vi "Sensor-Resistance-Sampling_withg_SMU1ar.vi"(1 "hold time (sec)":dbl=10.0 format="%#_13g", 2 "Gate step - extra milliseconds to wait":u32=20000, 3 "Current through sensor (A)":dbl format="%#_13g", 4 "Number of times measurement is done":i32=7, 6 "Number of heater steps":i32=7, 7 "Heater Step (V)":dbl=3.3) -> ()   [LabVIEW 2016]
uses:
  <vilib>/Utility/file.llb/Write To Spreadsheet File (DBL).vi
  <vilib>/Utility/file.llb/Read From Spreadsheet File (DBL).vi
  Driver/New driver/Agilent 415X Series.lvlib
panel:
  in  "Gate Step":dbl=-6.0
  in  "Gate Start":dbl format="%#_13g"
  in  "number of samples per heater step":i32=10
  out "error out":errorcluster
  out "Voltage across heater (VSU 1 and SMU4)":dbl[][](graph)
  out "Voltage measured between SMU1 (Common) and SMU2":dbl[](graph)
  out "SPA VISA resource name":refnum<visa-resource-name>
  in  "1. SPA VISA resource name":refnum<visa-resource-name>="GPIB0::14::INSTR"
  in  "error in (no error)":errorcluster
  # "2. Heater Parameters"
  # "3. Repeat Entire Cycle"
  # "4. Timings \n(Should be same as those when sampling Thermopower)"
  # "5. Other measurement parameters"
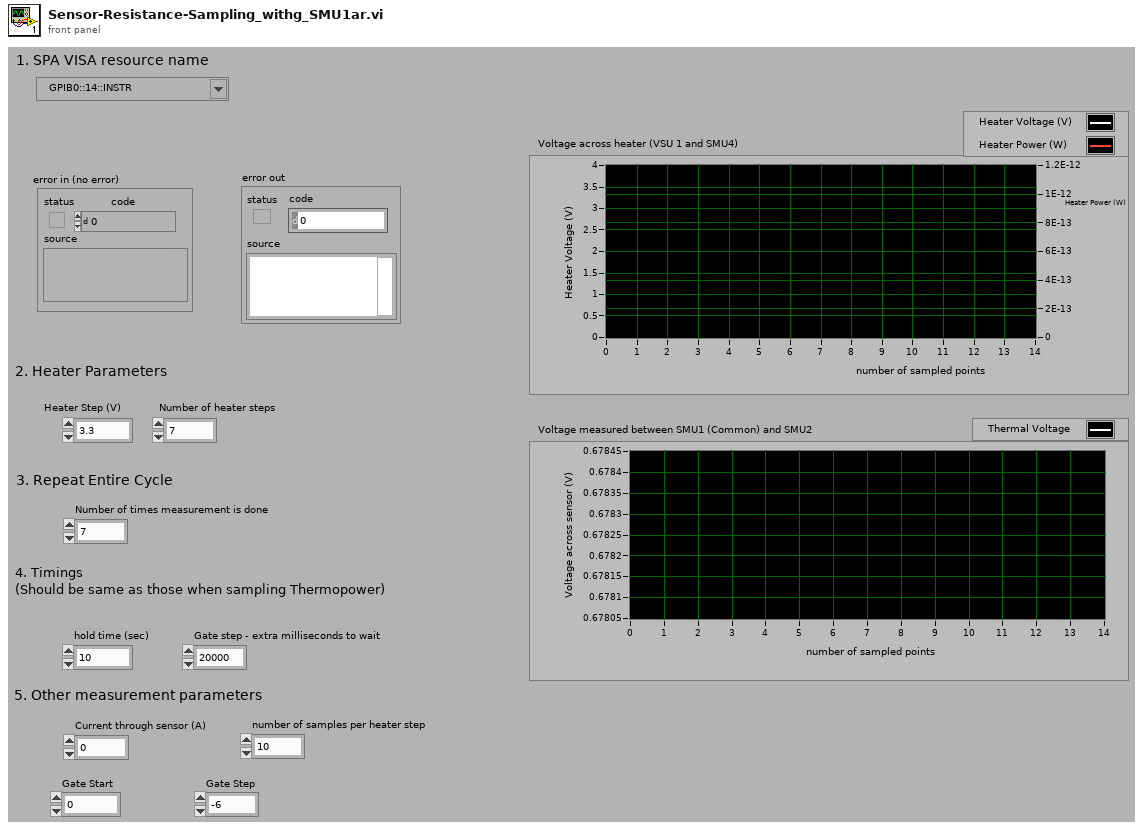
[diagram p1: front panel]
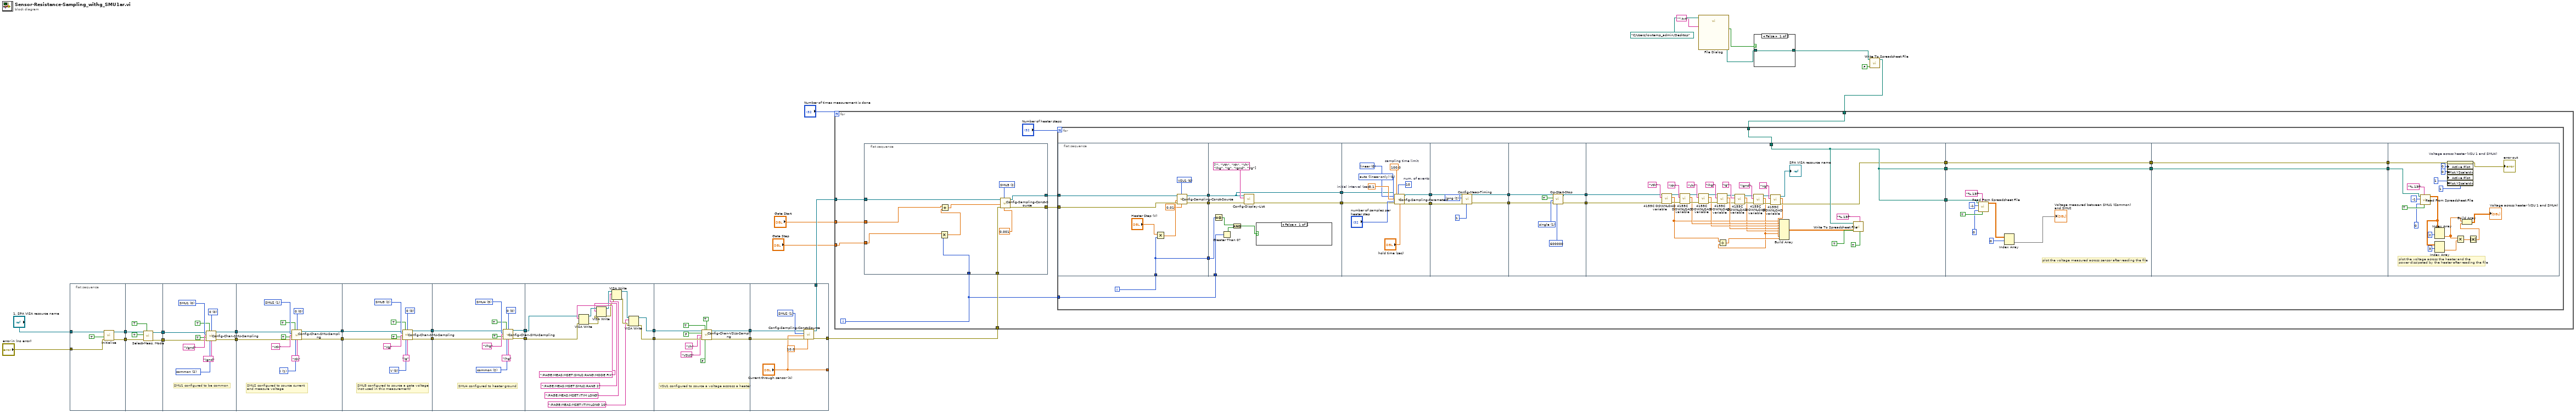
[diagram p0: block diagram]
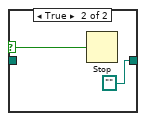
[diagram p2: hidden frame]
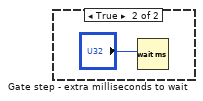
[diagram p3: hidden frame]
diagram:
  n1 = flat-sequence {
    tunnel: "error in (no error)" -> [w34]
    tunnel: "1. SPA VISA resource name" -> [w33]
    tunnel: [w32] -> w28
    tunnel: [w31] -> w27
    tunnel: w28 -> [w41]
    tunnel: w27 -> [w40]
    tunnel: [w37] -> w26
    tunnel: [w36] -> w25
    tunnel: w26 -> [w49]
    tunnel: w25 -> [w48]
    tunnel: [w47] -> w24
    tunnel: [w46] -> w23
    tunnel: w24 -> [w60]
    tunnel: w23 -> [w59]
    tunnel: [w58] -> w22
    tunnel: [w57] -> w21
    tunnel: w22 -> [w71]
    tunnel: w21 -> [w70]
    tunnel: [w69] -> w18
    tunnel: [w68] -> w17
    tunnel: w18 -> [w76]
    tunnel: [w77] -> w6
    tunnel: w17 -> [w75]
    tunnel: [w78] -> w4
    tunnel: w6 -> [w87]
    tunnel: [w88] -> w5
    tunnel: w4 -> [w86]
    tunnel: [w89] -> w3
    tunnel: w5 -> [w107]
    tunnel: w3 -> [w109]
    tunnel: [w108] -> w20
    tunnel: [w106] -> w19
    tunnel: w20 -> [w113]
    tunnel: w19 -> [w114]
    tunnel: [w112] -> w15
    tunnel: [w111] -> w14
    tunnel: ["Current through sensor (A)"] -> _
    frame #0 {
      n2 = call "Initialize.vi"("error in (no error)"=w34, "reset"=TRUE, "VISA resource name"=w33) -> ("error out"=w31:errorcluster, "VISA resource name out"=w32:refnum<visa-resource-name>)  [unwired: 2 in, 5 out]
    }
    frame #1 {
      n3 = call "Select-Meas. Mode.vi"("clear all channels"=TRUE, "error in (no error)"=w40, "measurement mode"=TRUE, "VISA resource name"=w41) -> ("error out"=w36:errorcluster, "VISA resource name out"=w37:refnum<visa-resource-name>)  [unwired: 1 in, 5 out]
    }
    frame #2 {
      w44 = 0 items=["0  ", "10K Ohms  ", "100K Ohms  ", "1M Ohms  "] ("series resistance *")
      w45 = 2 items=["V  ", "I  ", "  common  "] ("mode")
      w50 = 0 items=["SMU1  ", "SMU2  ", "SMU3  ", "SMU4  ", "SMU5  ", "SMU6  "] ("unit to configure")
      # "SMU1 configured to be common"
      n4 = call "Config-Chan-SMU-Sampling.vi"("VISA resource name in"=w49, "function"=TRUE, "series resistance *"=w44, "unit to configure"=w50, "V name (max 6 chars)"="Vgnd", "standby"=TRUE, "error in (no error)"=w48, "mode"=w45, "I name (max 6 chars)"="Ignd") -> ("VISA resource name out"=w47:refnum<visa-resource-name>, "error out"=w46:errorcluster)  [unwired: 5 out]
    }
    frame #3 {
      w54 = 0 items=["0  ", "10K Ohms  ", "100K Ohms  ", "1M Ohms  "] ("series resistance *")
      w56 = 1 items=["V  ", "I  ", "  common  "] ("mode")
      w61 = 1 items=["SMU1  ", "SMU2  ", "SMU3  ", "SMU4  ", "SMU5  ", "SMU6  "] ("unit to configure")
      # "SMU2 configured to source current \nand measure voltage"
      n5 = call "Config-Chan-SMU-Sampling.vi"("VISA resource name in"=w60, "function"=TRUE, "series resistance *"=w54, "unit to configure"=w61, "V name (max 6 chars)"="Vth", "standby"=TRUE, "error in (no error)"=w59, "mode"=w56, "I name (max 6 chars)"="Ith") -> ("VISA resource name out"=w58:refnum<visa-resource-name>, "error out"=w57:errorcluster)  [unwired: 5 out]
    }
    frame #4 {
      w65 = 0 items=["0  ", "10K Ohms  ", "100K Ohms  ", "1M Ohms  "] ("series resistance *")
      w67 = 0 items=["V  ", "I  ", "  common  "] ("mode")
      w72 = 2 items=["SMU1  ", "SMU2  ", "SMU3  ", "SMU4  ", "SMU5  ", "SMU6  "] ("unit to configure")
      # "SMU3 configured to source a gate voltage\n(not used in this measurement)"
      n6 = call "Config-Chan-SMU-Sampling.vi"("VISA resource name in"=w71, "function"=TRUE, "series resistance *"=w65, "unit to configure"=w72, "V name (max 6 chars)"="Vg", "standby"=TRUE, "error in (no error)"=w70, "mode"=w67, "I name (max 6 chars)"="Ig") -> ("VISA resource name out"=w69:refnum<visa-resource-name>, "error out"=w68:errorcluster)  [unwired: 5 out]
    }
    frame #5 {
      w80 = 0 items=["0  ", "10K Ohms  ", "100K Ohms  ", "1M Ohms  "] ("series resistance *")
      w82 = 2 items=["V  ", "I  ", "  common  "] ("mode")
      w83 = 3 items=["SMU1  ", "SMU2  ", "SMU3  ", "SMU4  ", "SMU5  ", "SMU6  "] ("unit to configure")
      # "SMU4 configured to heater ground"
      n7 = call "Config-Chan-SMU-Sampling.vi"("VISA resource name in"=w76, "function"=TRUE, "series resistance *"=w80, "unit to configure"=w83, "V name (max 6 chars)"="Vhg", "standby"=TRUE, "error in (no error)"=w75, "mode"=w82, "I name (max 6 chars)"="Ihg") -> ("VISA resource name out"=w77:refnum<visa-resource-name>, "error out"=w78:errorcluster)  [unwired: 5 out]
    }
    frame #6 {
      n8 = VISA Write(VISA resource name=w87, write buffer=":PAGE:MEAS:MSET:SMU2:RANG:MODE FIX", error in (no error)=w86) -> (VISA resource name out=w99:refnum<visa-resource-name>, error out=w98:errorcluster)  [unwired: 1 out]
      n9 = VISA Write(VISA resource name=w99, write buffer=":PAGE:MEAS:MSET:SMU2:RANG 2", error in (no error)=w98) -> (VISA resource name out=w94:refnum<visa-resource-name>, error out=w93:errorcluster)  [unwired: 1 out]
      n10 = VISA Write(VISA resource name=w94, write buffer=":PAGE:MEAS:MSET:ITIM LONG", error in (no error)=w93) -> (VISA resource name out=w92:refnum<visa-resource-name>, error out=w91:errorcluster)  [unwired: 1 out]
      n11 = VISA Write(VISA resource name=w92, write buffer=":PAGE:MEAS:MSET:ITIM:LONG 10", error in (no error)=w91) -> (VISA resource name out=w88:refnum<visa-resource-name>, error out=w89:errorcluster)  [unwired: 1 out]
    }
    frame #7 {
      # "VSU1 configured to source a voltage accross a heater"
      n12 = call "Config-Chan-VSUs-Sampling.vi"("VISA session"=w107, "VSU1 function"=TRUE, "VSU2 standby"=TRUE, "VSU1 standby"=FALSE, "VSU1 V name \n(max 6 chars)"="Vh" ("V name (max 6 chars)"), "VSU2 V name \n(max 6 chars)"="VSU2" ("V name (max 6 chars)"), "error in (no error)"=w109, "VSU2 function"=FALSE) -> ("VISA resource name out"=w106:refnum<visa-resource-name>, "error out"=w108:errorcluster)  [unwired: 6 out]
    }
    frame #8 {
      w115 = u16 1 items=["SMU 1", "SMU2", "SMU3", "SMU4", "SMU5", "SMU6", "VSU1", "VSU2"] ("unit (SMU1:0)")
      n13 = call "Config-Sampling-Const-Source.vi"("compliance (SMUs only)"=10.0, "error in (no error)"=w113, "source (V or A)"="Current through sensor (A)", "unit (SMU1:0)"=w115, "VISA session"=w114) -> ("error out"=w111:errorcluster, "VISA resource name out"=w112:refnum<visa-resource-name>)  [unwired: 5 out]
    }
  }
  n14 = call "File Dialog"("start path"=path "C:/Users/lowtemp_admin/Desktop", "pattern (all files)"="*.txt") -> ("selected path"=w12:path, "cancelled"=w11:bool)  [unwired: 10 in, 2 out]
  n15 = case shown="False" w11 {
    selector: w11 -> [_ w119]
    tunnel: w12 -> [w117 _]
    tunnel: [w117 path ""] -> w8
    frame False {
    }
    frame True {
      n16 = Stop(stop? (T)=w119) -> ()
    }
  }
  n17 = call-poly <vilib>:"Write To Spreadsheet File.vi"("append to file? (new file:F)"=FALSE, "file path (dialog if empty)"=w8) -> ("new file path (Not A Path if cancelled)"=w7:path)  [unwired: 6 in]
  n18 = for {
    N: "Number of times measurement is done" -> [_]
    tunnel: w15 -> [w125]
    tunnel: w14 -> [w124]
    tunnel: w7 -> [w123]
    tunnel: "Gate Start" -> [w122]
    tunnel: "Gate Step" -> [w121]
    i -> [w120]
    n19 = flat-sequence {
      tunnel: w120 -> [w266]
      tunnel: [w271] -> w127
      tunnel: [w270] -> w126
      tunnel: w125 -> [w269]
      tunnel: w124 -> [w268]
      tunnel: w122 -> [w263]
      tunnel: w121 -> [w262]
      frame #0 {
        w272 = u16 2 items=["SMU 1", "SMU2", "SMU3", "SMU4", "SMU5", "SMU6", "VSU1", "VSU2"] ("unit (SMU1:0)")
        n20 = Multiply(x=w262, y=w266) -> (x*y=w265:dbl)
        n21 = Add(x=w263, y=w265) -> (x+y=w264:dbl)
        n22 = call "Config-Sampling-Const-Source.vi"("compliance (SMUs only)"=0.001, "error in (no error)"=w268, "source (V or A)"=w264, "unit (SMU1:0)"=w272, "VISA session"=w269) -> ("error out"=w270:errorcluster, "VISA resource name out"=w271:refnum<visa-resource-name>)  [unwired: 5 out]
      }
    }
    n23 = for {
      N: "Number of heater steps" -> [_]
      tunnel: w127 -> [w140]
      tunnel: w126 -> [w139]
      tunnel: w123 -> [w138]
      tunnel: w120 -> [w131]
      i -> [w141]
      n24 = flat-sequence {
        tunnel: [w159] -> w151
        tunnel: [w158] -> w150
        tunnel: w141 -> [w153]
        tunnel: w140 -> [w157]
        tunnel: w139 -> [w156]
        tunnel: [w153] -> w132
        tunnel: w151 -> [w168]
        tunnel: w150 -> [w166]
        tunnel: [w167] -> w149
        tunnel: [w166] -> w148
        tunnel: w132 -> [w162]
        tunnel: w131 -> [w161]
        tunnel: w149 -> [w174]
        tunnel: w148 -> [w173]
        tunnel: [w172] -> w147
        tunnel: [w171] -> w146
        tunnel: w147 -> [w185]
        tunnel: w146 -> [w184]
        tunnel: [w183] -> w145
        tunnel: [w182] -> w144
        tunnel: w145 -> [w191]
        tunnel: w144 -> [w190]
        tunnel: [w189] -> w143
        tunnel: [w188] -> w142
        tunnel: w143 -> [w212]
        tunnel: w142 -> [w211]
        tunnel: w138 -> [w213]
        tunnel: [w213] -> w137
        tunnel: [w213] -> w136
        tunnel: [w201] -> w134
        tunnel: w137 -> [w237]
        tunnel: [w232] -> w130
        tunnel: w136 -> [w232]
        tunnel: w134 -> [w233]
        tunnel: [w233] -> w129
        tunnel: [w242] -> w135
        tunnel: [w241] -> w133
        tunnel: w129 -> [w241]
        tunnel: w130 -> [w242]
        tunnel: w135 -> [w243]
        tunnel: w133 -> [w248]
        frame #0 {
          w160 = u16 6 items=["SMU 1", "SMU2", "SMU3", "SMU4", "SMU5", "SMU6", "VSU1", "VSU2"] ("unit (SMU1:0)")
          n25 = Multiply(x="Heater Step (V)", y=w153) -> (x*y=w154:dbl)
          n26 = call "Config-Sampling-Const-Source.vi"("compliance (SMUs only)"=0.01, "error in (no error)"=w156, "source (V or A)"=w154, "unit (SMU1:0)"=w160, "VISA session"=w157) -> ("error out"=w159:errorcluster, "VISA resource name out"=w158:refnum<visa-resource-name>)  [unwired: 5 out]
        }
        frame #1 {
          n27 = Equal To 0?(x=w162) -> (x = 0?=w163:bool)
          n28 = Greater Than 0?(x=w161) -> (x > 0?=w164:bool)
          n29 = And(x=w163, y=w164) -> (x .and. y?=w165:bool)
          n30 = call "Config-Display-List.vi"("error in (no error)"=w168, "list (max 8 elements)"=string[] ["", "Vth", "Ith", "Vh", "Ihg", "Ig", "Ignd", "Vg"], "VISA session"=w166) -> ("error out"=w167:errorcluster)  [unwired: 1 in, 7 out]
          n31 = case shown="False" w165 {
            frame False {
            }
            frame True {
              n32 = Wait (ms)(milliseconds to wait="Gate step - extra milliseconds to wait") -> ()  [unwired: 1 out]
            }
          }
        }
        frame #2 {
          w175 = 100.0  # sampling time limit
          w176 = 0 items=["linear", "log 10", "log 25", "log 50", "thinned out"] ("mode (linear: 0)")
          w177 = 0 items=["auto (linear only)", "no limit", "set limit "] ("sampling time\n(linear/thinned-out only)")
          w178 = 0.1  # initial interval (sec)
          w179 = 10  # num. of events
          n33 = call "Config-Sampling-Parameters.vi"("VISA session"=w173, "mode (linear: 0)"=w176, "initial interval (sec)"=w178, "sampling time\n(linear/thinned-out only)"=w177, "number of samples"="number of samples per heater step", "error in (no error)"=w174, "sampling time limit"=w175, "num. of events"=w179, "hold time (sec)"="hold time (sec)") -> ("VISA resource name out"=w171:refnum<visa-resource-name>, "error out"=w172:errorcluster)  [unwired: 7 in, 10 out]
        }
        frame #3 {
          w187 = 2 items=["short  ", "medium  ", "long  "] ("integration time")
          n34 = call "Config-Meas-Timing.vi"("# PLCs for long integration time"=1, "error in (no error)"=w185, "integration time"=w187, "VISA session"=w184) -> ("error out"=w183:errorcluster, "VISA resource name out"=w182:refnum<visa-resource-name>)  [unwired: 2 in, 4 out]
        }
        frame #4 {
          w193 = 1 items=["stop  ", "single  ", "single-append  ", "stress start  ", "continuous  ", "standby on  ", "standby off  ", "zero  "] ("function (stop:0)")
          n35 = call "Op-Start-Stop.vi"("time to wait (30000ms)"=600000, "error in (no error)"=w191, "function (stop:0)"=w193, "wait until finish"=TRUE, "VISA resource name"=w190) -> ("error out"=w189:errorcluster, "VISA resource name out"=w188:refnum<visa-resource-name>)  [unwired: 5 out]
        }
        frame #5 {
          n36 = call "4155C DOWNLOAD variable.vi"("error in (no error)"=w212, "Variable name"="Vth", "VISA resource name in"=w211) -> ("error out"=w221:errorcluster, "Output data"=w198:dbl[], "VISA Resource Name out"=w224:refnum<visa-resource-name>)  [unwired: 2 out]
          n37 = call "4155C DOWNLOAD variable.vi"("error in (no error)"=w221, "Variable name"="Ith", "VISA resource name in"=w224) -> ("error out"=w220:errorcluster, "Output data"=w218:dbl[], "VISA Resource Name out"=w223:refnum<visa-resource-name>)  [unwired: 2 out]
          n38 = call "4155C DOWNLOAD variable.vi"("error in (no error)"=w220, "Variable name"="Vh", "VISA resource name in"=w223) -> ("error out"=w219:errorcluster, "Output data"=w217:dbl[], "VISA Resource Name out"=w222:refnum<visa-resource-name>)  [unwired: 2 out]
          n39 = call "4155C DOWNLOAD variable.vi"("error in (no error)"=w219, "Variable name"="Ihg", "VISA resource name in"=w222) -> ("error out"=w206:errorcluster, "Output data"=w216:dbl[], "VISA Resource Name out"=w205:refnum<visa-resource-name>)  [unwired: 2 out]
          n40 = call "4155C DOWNLOAD variable.vi"("error in (no error)"=w206, "Variable name"="Ig", "VISA resource name in"=w205) -> ("error out"=w208:errorcluster, "Output data"=w196:dbl[], "VISA Resource Name out"=w209:refnum<visa-resource-name>)  [unwired: 2 out]
          n41 = call "4155C DOWNLOAD variable.vi"("error in (no error)"=w208, "Variable name"="Ignd", "VISA resource name in"=w209) -> ("error out"=w202:errorcluster, "Output data"=w195:dbl[], "VISA Resource Name out"=w203:refnum<visa-resource-name>)  [unwired: 2 out]
          n42 = Divide(x=w198, y=w195) -> (x/y=w197:dbl[])
          n43 = call "4155C DOWNLOAD variable.vi"("error in (no error)"=w202, "Variable name"="Vg", "VISA resource name in"=w203) -> ("error out"=w201:errorcluster, "Output data"=w199:dbl[], "VISA Resource Name out"=→"SPA VISA resource name":refnum<visa-resource-name>)  [unwired: 2 out]
          n44 = Build Array(w198, w218, w217, w216, w196, w195, w199, w197) -> (w215:dbl[][])
          n45 = call-poly <vilib>:"Write To Spreadsheet File.vi"("transpose? (no:F)"=TRUE, "format (%.3f)"="%.13f", "append to file? (new file:F)"=TRUE, "2D data"=w215, "file path (dialog if empty)"=w213) -> ()  [unwired: 1 in, 3 out]
        }
        frame #6 {
          # "plot the voltage measured across sensor after reading the file"
          n46 = call-poly <vilib>:"Read From Spreadsheet File.vi"("transpose (no:F)"=TRUE, "format (%.3f)"="%.13f", "max characters/row  (no limit:0)"=0, "number of rows (all:-1)"=-1, "file path (dialog if empty)"=w237) -> ("all rows"=w234:dbl[][])  [unwired: 6 out]
          n47 = Index Array(array=w234, index (row)=0) -> (element=→"Voltage measured between SMU1 (Common) and SMU2":dbl[])  [unwired: 1 in]
        }
        frame #7 {
        }
        frame #8 {
          # "plot the voltage across the heater and the \npower dissipated by the heater after reading the file"
          n48 = call-poly <vilib>:"Read From Spreadsheet File.vi"("transpose (no:F)"=TRUE, "format (%.3f)"="%.13f", "max characters/row  (no limit:0)"=0, "number of rows (all:-1)"=-1, "file path (dialog if empty)"=w243) -> ("all rows"=w256:dbl[][])  [unwired: 6 out]
          n49 = Index Array(array=w256, index (row)=2) -> (element=w250:dbl[])  [unwired: 1 in]
          n50 = Index Array(array=w256, index (row)=3) -> (element=w254:dbl[])  [unwired: 1 in]
          n51 = property on="Voltage across heater (VSU 1 and SMU4)" class="WFGraph (strict)"(error in=w248, "Active Plot"=u32 0, "Plot.YScaleIdx"=u32 0 ("Plot.Y Scale Index"), "Active Plot"=u32 1, "Plot.YScaleIdx"=u32 1 ("Plot.Y Scale Index")) -> (error out=→"error out":errorcluster)  [unwired: 1 in, 1 out]
          n52 = Multiply(x=w250, y=w254) -> (x*y=w253:dbl[])
          n53 = Absolute Value(x=w253) -> (abs(x)=w252:dbl[])
          n54 = Build Array(w250, w252) -> (→"Voltage across heater (VSU 1 and SMU4)":dbl[][])
        }
      }
    }
  }
